vi "test Read Double Array.vi"(8 "error in (no error)":errorcluster, 11 "TestCase in":refnum<class "Buffer Tests.lvclass">=refnum) -> (0 "error out":errorcluster, 3 "TestCase out":refnum<class "Buffer Tests.lvclass">)   [LabVIEW 2021, in "Buffer Tests.lvclass"]
uses:
  Buffer Tests.lvclass
  Classes/Buffer/Buffer.lvclass
  Classes/Buffer/Read Buffer 1D DBL.vi
  <vilib>/NI/Memory Manager/Classes/Pointer/Pointer.lvclass
  C:/Program Files/National Instruments/LabVIEW 2021/vi.lib/NI/Memory Manager/Classes/Pointer/Pointer.lvclass
  C:/dev/git/custom-devices/niveristand-data-sharing-framework-custom-device/Source/Core/Classes/Buffer/Buffer.lvclass
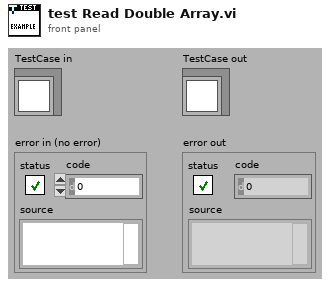
[diagram p1: front panel]
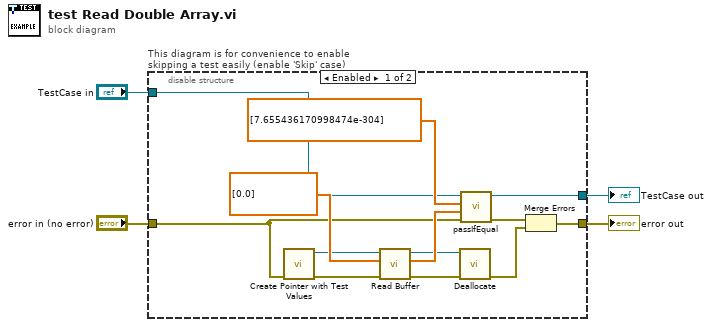
[diagram p0: block diagram]
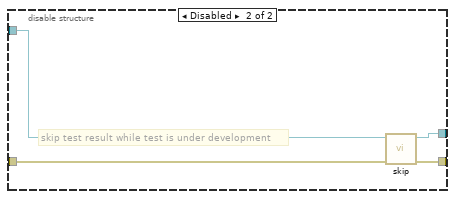
[diagram p2: hidden frame]
diagram:
  n1 = disable-structure "This diagram is for convenience to enable skipping a test easily (enable 'Skip' case)" shown="Enabled" {
    disable-tunnel: "TestCase in" -> [w10 w21]
    disable-tunnel: [w16 w19] -> w1
    disable-tunnel: [w14 w20] -> w3
    disable-tunnel: "error in (no error)" -> [w7 w18]
    frame Enabled {
      n2 = call "Create Pointer with Test Values.vi"("error in (no error)"=w7) -> ("error out"=w8:errorcluster, "Buffer out"=w9:refnum<class "Buffer.lvclass">)  [unwired: 9 in]
      n3 = call-poly "Read Buffer.vi"("error in (no error)"=w8, "dst array in"=dbl[] [0.0] ("buffer in"), "Buffer in"=w9) -> ("error out"=w13:errorcluster, "dst array out"=w12:dbl[], "Buffer out"=w5:refnum<class "Buffer.lvclass">)  [unwired: 5 in, 1 out]
      n4 = call <vilib>:"Deallocate.vi"("error in (no error)"=w13, "Pointer"=w5) -> ("error out"=w6:errorcluster)  [unwired: 8 in, 1 out]
      n5 = call-dynamic "passIfEqual.vi"("error in (no error)"=w7, "y"=w12, "x"=dbl[] [7.655436170998474e-304] ("*(type *) &x 2"), "TestCase in"=w10) -> ("error out"=w15:errorcluster, "TestCase out"=w16:refnum<class "Buffer Tests.lvclass">)  [unwired: 6 in]
      n6 = Merge Errors(w15, w6) -> (w14:errorcluster)
    }
    frame Disabled {
      # "skip test result while test is under development"
      n7 = call <vilib>:"skip.vi"("error in (no error)"=w18, "TestCase in"=w21) -> ("error out"=w20:errorcluster, "TestCase out"=w19:refnum<class "Buffer Tests.lvclass">)  [unwired: 8 in]
    }
  }
  "error out" <- w3
  "TestCase out" <- w1
